vi "TCP Ping.vi"(8 "error in (no error)":errorcluster, 10 "timeout(100)":i32=100, 11 "hostNameOrAddress":string="127.0.0.1") -> (0 "error out":errorcluster, 2 "Status":i32(ring) items=["Success"=0, "DestinationNetworkUnreachable"=11002, "DestinationHostUnreachable"=11003, "DestinationProhibited, DestinationProtocolUnreachable"=11004, "DestinationPortUnreachable"=11005, "NoResources"=11006, "BadOption"=11007, "HardwareError"=11008, "PacketTooBig"=11009, "TimedOut"=11010, "BadRoute"=11012, "TtlExpired"=11013, "TtlReassemblyTimeExceeded"=11014, "ParameterProblem"=11015, "SourceQuench"=11016, "BadDestination"=11018, "DestinationUnreachable"=11040, "TimeExceeded"=11041, "BadHeader"=11042, "UnrecognizedNextHeader"=11043, "IcmpError"=11044, "DestinationScopeMismatch"=11045, "Unknown"=-1])   [LabVIEW 2014, in "FileSync -- Base.lvlib" / "Protocol.lvclass"]
uses:
  Protocol.lvclass
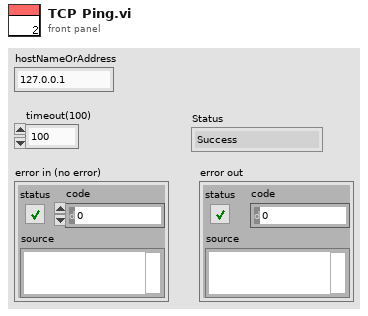
[diagram p1: front panel]
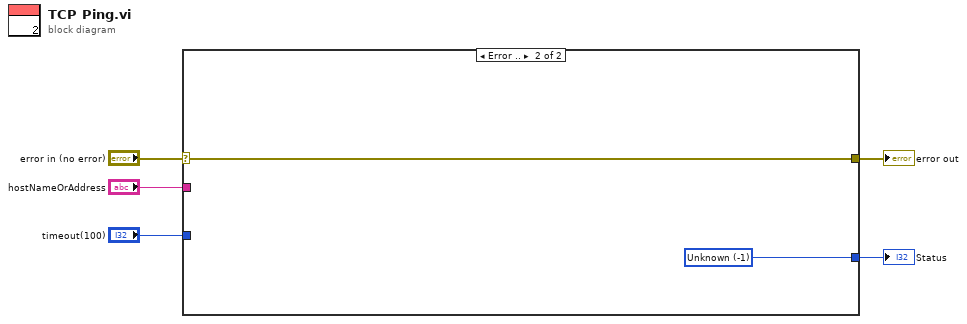
[diagram p0: block diagram]
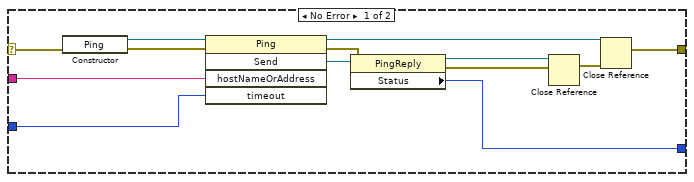
[diagram p2: hidden frame]
diagram:
  n1 = case shown="Error .." "error in (no error)" {
    selector: "error in (no error)" -> [w17 w20]
    tunnel: [w18 w20] -> w5
    tunnel: [w10 w19] -> w3
    tunnel: "hostNameOrAddress" -> [w8 _]
    tunnel: "timeout(100)" -> [w6 _]
    frame No Error {
      n2 = constructor class="Ping" ("Constructor Node")(error in=w17) -> (reference out=w9:refnum<k24>, error out=w13:errorcluster)  [unwired: 2 in, 1 out]
      n3 = invoke on="Invoke Node" class="Ping" method="Send"(reference=w9, error in=w13, "hostNameOrAddress"=w8, "timeout"=w6) -> (reference out=w12:refnum<k24>, error out=w14:errorcluster, "Send"=w7:refnum<k24>)  [unwired: 1 in, 2 out]
      n4 = property on="Property Node" class="PingReply"(reference=w7, error in=w14) -> (reference out=w11:refnum<k24>, error out=w15:errorcluster, "Status"=w10:i32)
      n5 = Close Reference(reference=w11, error in (no error)=w15) -> (error out=w16:errorcluster)
      n6 = Close Reference(reference=w12, error in (no error)=w16) -> (error out=w18:errorcluster)
    }
    frame Error {
      w19 = -1 items=["Success"=0, "DestinationNetworkUnreachable"=11002, "DestinationHostUnreachable"=11003, "DestinationProhibited, DestinationProtocolUnreachable"=11004, "DestinationPortUnreachable"=11005, "NoResources"=11006, "BadOption"=11007, "HardwareError"=11008, "PacketTooBig"=11009, "TimedOut"=11010, "BadRoute"=11012, "TtlExpired"=11013, "TtlReassemblyTimeExceeded"=11014, "ParameterProblem"=11015, "SourceQuench"=11016, "BadDestination"=11018, "DestinationUnreachable"=11040, "TimeExceeded"=11041, "BadHeader"=11042, "UnrecognizedNextHeader"=11043, "IcmpError"=11044, "DestinationScopeMismatch"=11045, "Unknown"=-1] ("Status")
    }
  }
  "error out" <- w5
  "Status" <- w3
